vi "Configure Sweep Characteristic.vi"(4 "Auto Gating Marker (0)":dbl, 5 "Reference (1: Reference 1)":i32(ring)=1 items=["Reference 1"=1, "Reference 2"=2], 6 "Auto Gating (F: Disable)":bool, 7 "Sweep Delay (0 s)":dbl, 8 "error in (no error)":errorcluster, 9 "Time-gated Period (0.0001 s)":dbl=0.0001, 10 "Gate (1: Gate 1)":i32(ring)=1 items=["Gate 1"=1, "Gate 2"=2, "Gate 3"=3, "Gate 4"=4], 11 "VISA resource name":refnum<visa-resource-name>) -> (0 "error out":errorcluster, 3 "VISA resource name out":refnum<visa-resource-name>)   [LabVIEW 2018, in "Agilent U2000 Series.lvlib"]
doc: "Changes the configurations for sweep mode.\n\nNote:\nThis VI is only applicable for Agilent U2021/2XA and U2042XA/U2044XA/U2049XA models."
uses:
  Agilent U2000 Series.lvlib
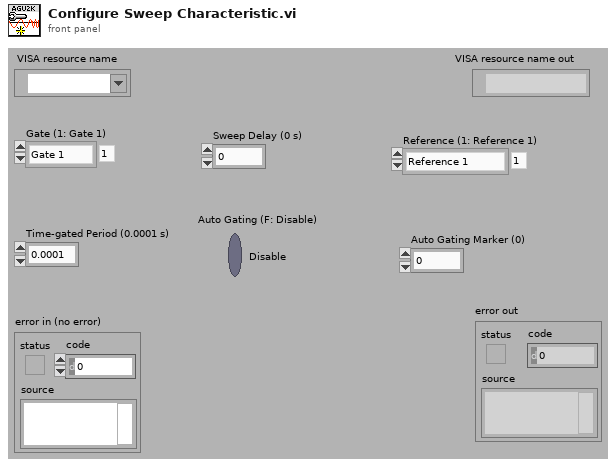
[diagram p1: front panel]
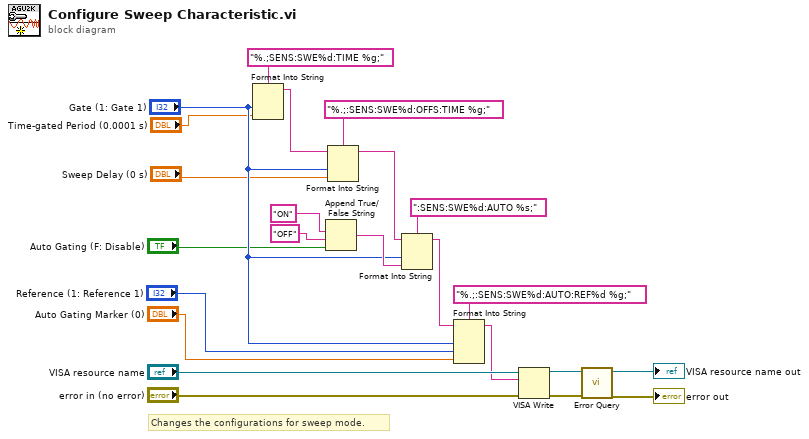
[diagram p0: block diagram]
diagram:
  # "Changes the configurations for sweep mode."
  n1 = Format Into String(format string="%.;SENS:SWE%d:TIME %g;", "Gate (1: Gate 1)", "Time-gated Period (0.0001 s)") -> (resulting string=w23:string)  [unwired: 2 in, 1 out]
  n2 = Append True/False String(1:"Auto Gating (F: Disable)", 2:"OFF", 3:"ON") -> (0:w19:string)  [unwired: 1 out]
  n3 = Format Into String(format string="%.;:SENS:SWE%d:OFFS:TIME %g;", initial string=w23, "Gate (1: Gate 1)", "Sweep Delay (0 s)") -> (resulting string=w17:string)  [unwired: 1 in, 1 out]
  n4 = Format Into String(format string=":SENS:SWE%d:AUTO %s;", initial string=w17, "Gate (1: Gate 1)", w19) -> (resulting string=w18:string)  [unwired: 1 in, 1 out]
  n5 = Format Into String(format string="%.;:SENS:SWE%d:AUTO:REF%d %g;", initial string=w18, "Gate (1: Gate 1)", "Reference (1: Reference 1)", "Auto Gating Marker (0)") -> (resulting string=w1:string)  [unwired: 1 in, 1 out]
  n6 = VISA Write(VISA resource name="VISA resource name", write buffer=w1, error in (no error)="error in (no error)") -> (VISA resource name out=w7:refnum<visa-resource-name>, error out=w6:errorcluster)  [unwired: 1 out]
  n7 = call "Error Query.vi"("error in (no error)"=w6, "VISA resource name"=w7) -> ("error out"=→"error out":errorcluster, "VISA resource name out"=→"VISA resource name out":refnum<visa-resource-name>)  [unwired: 8 out]
